vi "PH_SRDG645.ProcEvents.vi"(0 "i ref in":refnum<vi>, 5 "error in":errorcluster) -> (14 "i ref out":refnum<vi>, 19 "error out":errorcluster)   [LabVIEW 2014, in "PH_SRDG645.lvlib"]
doc: "This method is used to define the events the object will listen to. Add your own events here."
uses:
  PH_SRDG645.lvlib
  CSCore/BaseProcess/BaseProcess.event definition.ctl
  CSCore/CAEObj/CAEObj.event definition.ctl
  CSCore/BaseProcess/BaseProcess.descriptor string definition.ctl
  CSCore/BaseProcess/BaseProcess.lvlib
  CSCore/CAEObj/CAEObj.lvlib
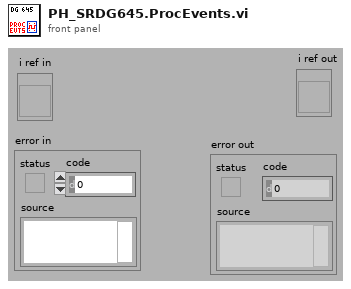
[diagram p1: front panel]
types:
  T1 = typedef "BaseProcess.lvlib/BaseProcess.event definition.ctl" = cluster{"CAEEvtDef":T2, "Data Descriptor":T3}
  T2 = typedef "CAEObj.lvlib/CAEObj.event definition.ctl" = cluster{"URL":string, "enable":bool, "ignoreResID":bool}
  T3 = typedef "BaseProcess.lvlib/BaseProcess.descriptor string definition.ctl" = string
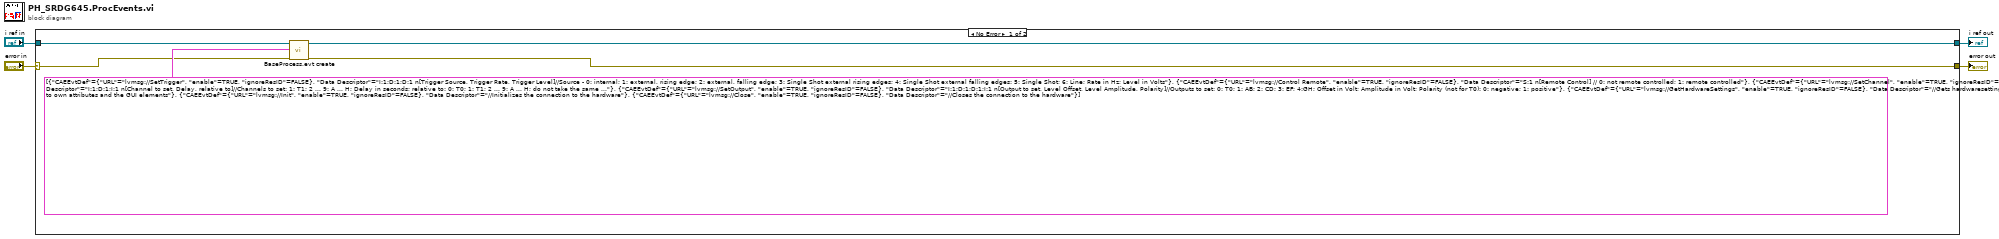
[diagram p0: block diagram]
diagram:
  n1 = case shown="No Error" "error in" {
    selector: "error in" -> [w5 w11]
    tunnel: "i ref in" -> [w9 w10]
    tunnel: [w8 w11] -> w3
    tunnel: [w7 w10] -> w2
    frame No Error {
      n2 = call "BaseProcess.evt create.vi"("i ref in"=w9, "newEvents"=T1[] [{"CAEEvtDef"={"URL"="lvmsg://SetTrigger", "enable"=TRUE, "ignoreResID"=FALSE}, "Data Descriptor"="I:1;D:1;D:1 n[Trigger Source, Trigger Rate, Trigger Level]//Source - 0: internal; 1: external, rising edge; 2: external, falling edge; 3: Single Shot external rising edges; 4: Single Shot external falling edges: 5: Single Shot; 6: Line; Rate in Hz; Level in Volts"}, {"CAEEvtDef"={"URL"="lvmsg://Control Remote", "enable"=TRUE, "ignoreResID"=FALSE}, "Data Descriptor"="S:1 n[Remote Control] // 0: not remote controlled; 1: remote controlled"}, {"CAEEvtDef"={"URL"="lvmsg://SetChannel", "enable"=TRUE, "ignoreResID"=FALSE}, "Data Descriptor"="I:1;D:1;I:1 n[Channel to set, Delay, relative to]//Channels to set: 1: T1; 2 ... 9: A ... H; Delay in seconds; relative to: 0: T0; 1: T1; 2 ... 9: A ... H; do not take the same ..."}, {"CAEEvtDef"={"URL"="lvmsg://SetOutput", "enable"=TRUE, "ignoreResID"=FALSE}, "Data Descriptor"="I:1;D:1;D:1;I:1 n[Output to set, Level Offset, Level Amplitude, Polarity]//Outputs to set: 0: T0; 1: AB; 2: CD; 3: EF; 4:GH; Offset in Volt; Amplitude in Volt; Polarity (not for T0): 0: negative; 1: positive"}, {"CAEEvtDef"={"URL"="lvmsg://GetHardwareSettings", "enable"=TRUE, "ignoreResID"=FALSE}, "Data Descriptor"="//Gets hardwaresettings and sets them to own attributes and the GUI elements"}, {"CAEEvtDef"={"URL"="lvmsg://Init", "enable"=TRUE, "ignoreResID"=FALSE}, "Data Descriptor"="//Initializes the connection to the hardware"}, {"CAEEvtDef"={"URL"="lvmsg://Close", "enable"=TRUE, "ignoreResID"=FALSE}, "Data Descriptor"="//Closes the connection to the hardware"}] ("new events"), "error in (no error)"=w5) -> ("i ref out"=w7:refnum<vi>, "error out"=w8:errorcluster)  [unwired: 13 in, 2 out]
    }
    frame Error {
    }
  }
  "i ref out" <- w2
  "error out" <- w3
